vi "CalCheckRatios.vi"() -> (5 "Plug in titles":string[](array[string]), 7 "Plug in values":string[](array[string]))   [LabVIEW 2011]
uses:
  Globals/Meas_global.vi
panel:
  out "subarray 2":string[](array[string])
  out "subarray":string[](array[string])
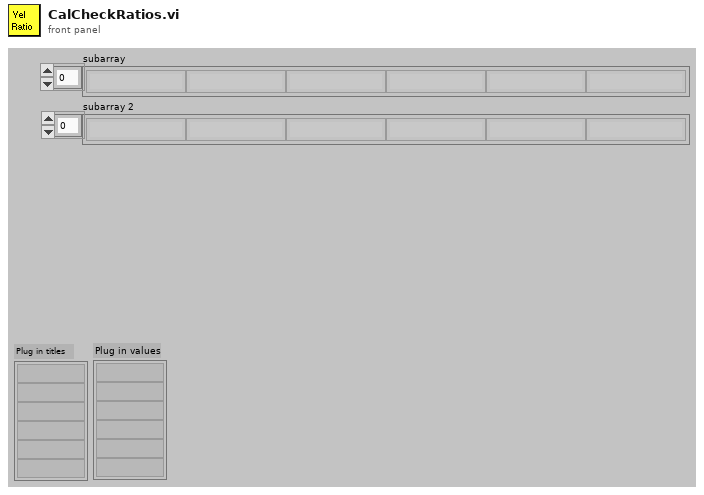
[diagram p1: front panel]
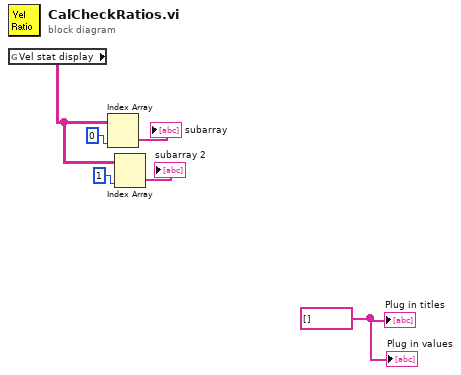
[diagram p0: block diagram]
diagram:
  w6 = string[] [] ("Plug in titles")
  n1 = global read "Meas_global.vi" "Vel stat display"() -> (w5:string[][])
  n2 = Index Array(array=w5, index (col)=0 ("index")) -> (element=→"subarray":string[])  [unwired: 1 in]
  n3 = Index Array(array=w5, index (col)=1 ("index")) -> (element=→"subarray 2":string[])  [unwired: 1 in]
  "Plug in values" <- w6
  "Plug in titles" <- w6
